vi "create_tasks.vi"(8 "error in":errorcluster, 11 "GenericPlugin in":refnum<class "ClockDL100201DAQmx.lvclass">) -> (0 "error out":errorcluster, 3 "GenericPlugin out":refnum<class "ClockDL100201DAQmx.lvclass">)   [LabVIEW 2010, in "ClockDL100201DAQmx.lvclass"]
uses:
  ClockDL100201DAQmx.lvclass
  ClockDL100201DAQmx.lvclass/ClockDL100201DAQmx.ctl
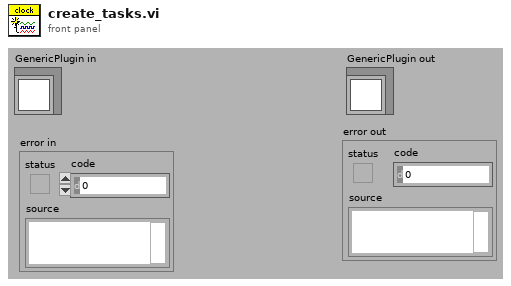
[diagram p1: front panel]
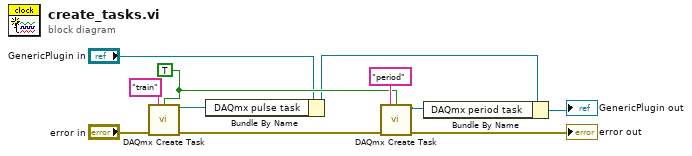
[diagram p0: block diagram]
diagram:
  w10 = TRUE ("auto cleanup")
  n1 = call <vilib>:"DAQmx Create Task.vi"("new task name"="train", "auto cleanup"=w10, "error in"="error in") -> ("task out"=w2:refnum<k21>, "error out"=w1:errorcluster)  [unwired: 11 in]
  n2 = Bundle By Name(cluster="GenericPlugin in", "DAQmx pulse task"=w2) -> (w7:refnum<class "ClockDL100201DAQmx.lvclass">)
  n3 = call <vilib>:"DAQmx Create Task.vi"("new task name"="period", "auto cleanup"=w10, "error in"=w1) -> ("task out"=w3:refnum<k21>, "error out"=→"error out":errorcluster)  [unwired: 11 in]
  n4 = Bundle By Name(cluster=w7, "DAQmx period task"=w3) -> (→"GenericPlugin out":refnum<class "ClockDL100201DAQmx.lvclass">)
